vi "SetNullPointOffset.vi"(0 "handle in":i32, 1 "UnitAddress(0)":u16, 2 "MotNr(0)":u8, 5 "error in":errorcluster, 7 "NullOffset(0)":i32, 9 "TestNullRange(240)":u16=240) -> (14 "handle out":i32, 19 "error out":errorcluster)   [LabVIEW 2014, in "Sixpack - Driver.lvlib"]
doc: "Der Referenzpunkt-Offset legt den Referenzpunkt auf die angegebene Position. Wird dieser Befehl nicht verwendet ist der Referenzpunkt identisch mit dem Nullpunkt. Es handelt sich nur um eine Koordinatentransformation, die am Verhalten der Referenzfahrten nichts ändert. Sie kann z.B. genutzt werden, um den Nullpunkt an das Ende des Fahrbereichs zu verlegen, etwa bei Referenzpunkten in der Mitte einer Fahrstrecke, um dann nur mit positiven Koordinaten arbeiten zu müssen. Siehe auch Kapitel 3.4.3. Wenn gleichzeitig der Test auf zu frühes Unterbrechen des Referenzschalters (siehe Befehl SetMotorParameters, Flag MT_STOPNULL) eingeschaltet ist, kann über die Variable TestNullRange ein kleiner Bereich um den Referenzpunkt herum vom Test ausgenommen werden. Außerhalb dieses Bereiches werden bei Fahrt auf den Referenzpunkt über den Referenzschalter ein Nothalt und eine anschließende Referenzfahrt ausgelöst. Siehe auch Kapitel 3.4.5.\n\nCMD $18\nMotorNr (0...5)\nNullOffset (signed long): Distanz zwischen Nullpunkt und Referenzschalter\nTestNullRange (0..65535): Bereich in dem Nullschalter aktiv sein darf"
uses:
  Sixpack - Driver.lvlib
  DLL/PackDLL.dll
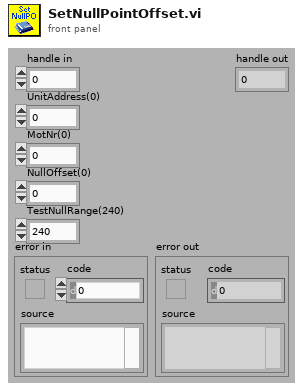
[diagram p1: front panel]
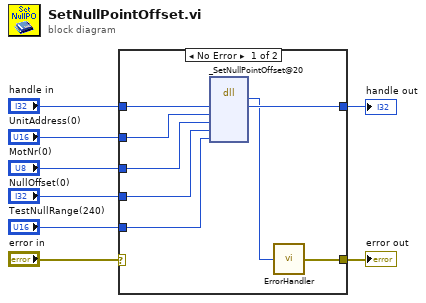
[diagram p0: block diagram]
diagram:
  n1 = case shown="No Error" "error in" {
    selector: "error in" -> [_ w17]
    tunnel: "handle in" -> [w16 w18]
    tunnel: [w15 w18] -> w7
    tunnel: "UnitAddress(0)" -> [w14 _]
    tunnel: "MotNr(0)" -> [w13 _]
    tunnel: "NullOffset(0)" -> [w12 _]
    tunnel: "TestNullRange(240)" -> [w11 _]
    tunnel: [w9 w17] -> w2
    frame No Error {
      n2 = dll-call lib="D:/CS-Source/LV2014/GPL/instr.lib/SixPack/PackDLL/DLL/PackDLL.dll" fn="_SetNullPointOffset@20" label="SetNullPointOffset"("HANDLE"=w16, "UnitAddress"=w14, "MotNr"=w13, "NullOffset"=w12, "TestNullRange"=w11) -> ("BOOLEAN"=w10:i8, "HANDLE"=w15:i32)  [unwired: 7 in, 2 out]
      n3 = call "ErrorHandler.vi"("BOOLEAN"=w10) -> ("error out"=w9:errorcluster)
    }
    frame Error {
    }
  }
  "handle out" <- w7
  "error out" <- w2
